vi "Post-Install Custom Action - Platform Specific PPLs.vi"(10 "Variant":variant) -> (0 "error out":errorcluster)   [LabVIEW 2020]
uses:
  <vilib>/Utility/lvfile.llb/FT_FileTypes.ctl
  <vilib>/Utility/lvfile.llb/NI_FileType.lvlib
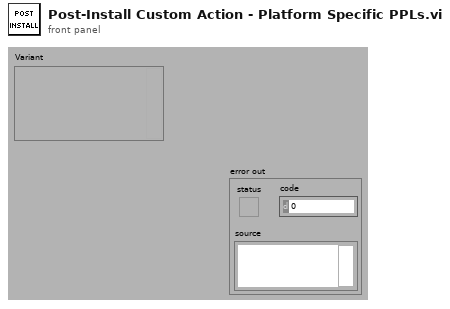
[diagram p1: front panel]
types:
  T1 = typedef "NI_FileType.lvlib/FT_FileTypes.ctl" = enum32{"Invalid file/path", "Unknown type", "Instrument", "Control", "Polymorphic VI", "Project", "Library", "LVClass", "XControl", "XNode", "CIN", "Run-time menu", "Palette menu", "LLB", "Shortcut", "Directory", "Class Private Data Control", "Statechart", "MathScript .m file", "Ladder Diagram", "LVLibp"}
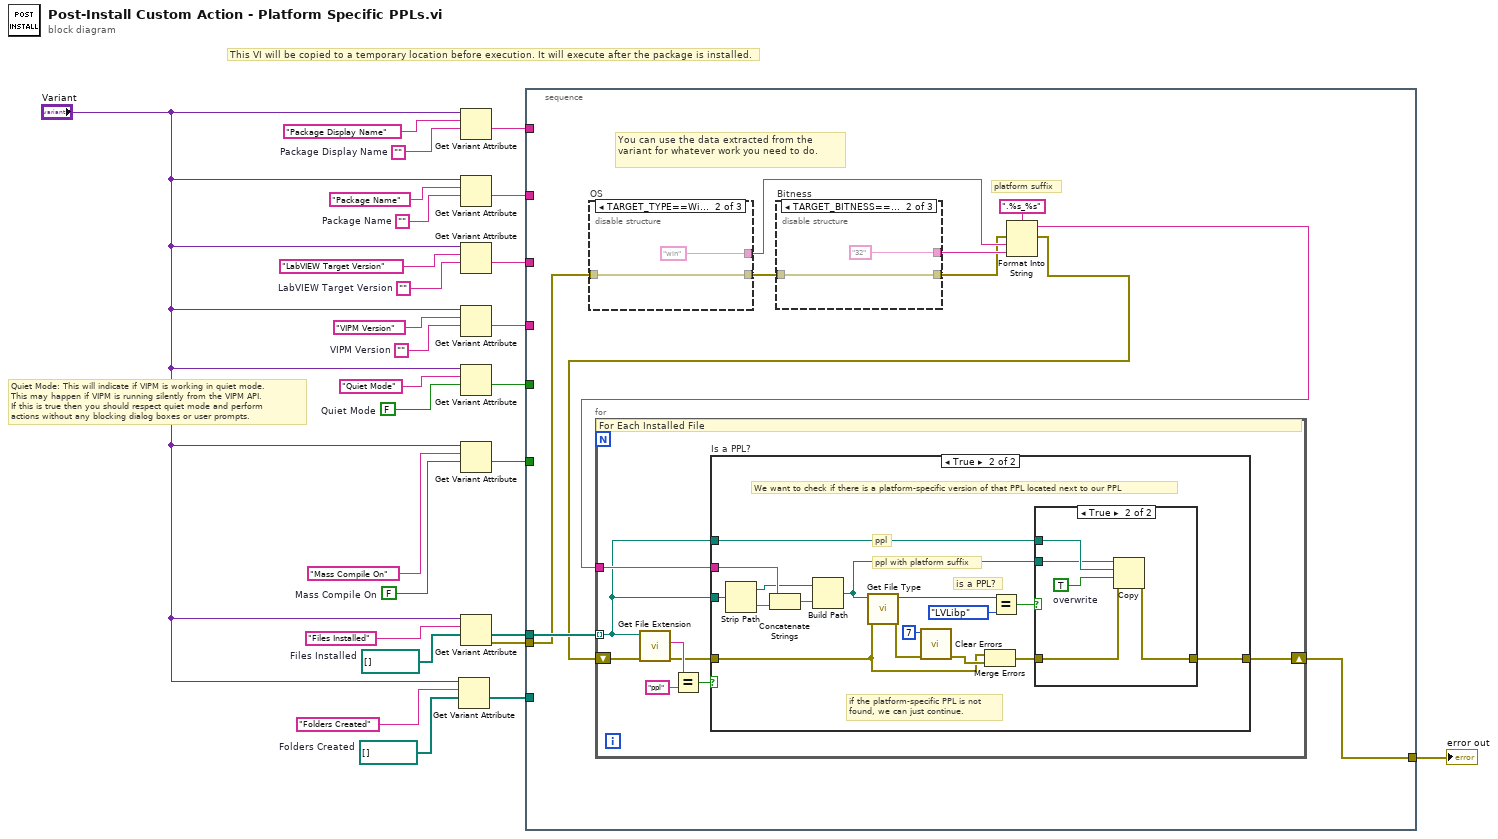
[diagram p0: block diagram]
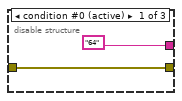
[diagram p2: hidden frame]
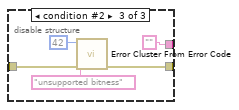
[diagram p3: hidden frame]
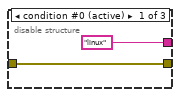
[diagram p4: hidden frame]
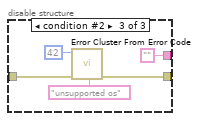
[diagram p5: hidden frame]
diagram:
  w3 = path[] []  # Folders Created
  w4 = path[] []  # Files Installed
  w10 = FALSE  # Mass Compile On
  w11 = ""  # Package Display Name
  w18 = FALSE  # Quiet Mode
  w21 = ""  # VIPM Version
  w23 = ""  # LabVIEW Target Version
  w25 = ""  # Package Name
  # "Quiet Mode: This will indicate if VIPM is working in quiet mode.\nThis may happen if VIPM is running silently from the VIPM API.\nIf this is true then you should respect quiet mode and perform\nactions without any blocking dialog boxes or user prompts."
  # "This VI will be copied to a temporary location before execution. It will execute after the package is installed."
  n1 = Get Variant Attribute(Variant="Variant", name="Folders Created", default value (empty Variant)=w3) -> (value=w8:path[])  [unwired: 1 in, 3 out]
  n2 = Get Variant Attribute(Variant="Variant", name="Package Display Name", default value (empty Variant)=w11) -> (value=w17:string)  [unwired: 1 in, 3 out]
  n3 = Get Variant Attribute(Variant="Variant", name="Package Name", default value (empty Variant)=w25) -> (value=w16:string)  [unwired: 1 in, 3 out]
  n4 = Get Variant Attribute(Variant="Variant", name="LabVIEW Target Version", default value (empty Variant)=w23) -> (value=w15:string)  [unwired: 1 in, 3 out]
  n5 = Get Variant Attribute(Variant="Variant", name="VIPM Version", default value (empty Variant)=w21) -> (value=w14:string)  [unwired: 1 in, 3 out]
  n6 = Get Variant Attribute(Variant="Variant", name="Quiet Mode", default value (empty Variant)=w18) -> (value=w13:bool)  [unwired: 1 in, 3 out]
  n7 = Get Variant Attribute(Variant="Variant", name="Mass Compile On", default value (empty Variant)=w10) -> (value=w12:bool)  [unwired: 1 in, 3 out]
  n8 = Get Variant Attribute(Variant="Variant", name="Files Installed", default value (empty Variant)=w4) -> (value=w7:path[], error out=w2:errorcluster)  [unwired: 1 in, 2 out]
  n9 = stacked-sequence {
    tunnel: w17 -> [_]
    tunnel: w16 -> [_]
    tunnel: w15 -> [_]
    tunnel: w14 -> [_]
    tunnel: w13 -> [_]
    tunnel: w12 -> [_]
    tunnel: w7 -> [w37]
    tunnel: w8 -> [_]
    tunnel: w2 -> [w35]
    tunnel: [w30] -> w1
    frame #0 {
      # "platform suffix"
      # "You can use the data extracted from the variant for whatever work you need to do."
      n10 = disable-structure "OS" shown="TARGET_TYPE==Windows" {
        disable-tunnel: ["linux" "win" ""] -> w34
        disable-tunnel: [w47 w49 w52] -> w36
        disable-tunnel: w35 -> [w47 w49 w51]
        frame condition #0 (active) {
        }
        frame condition #1 {
        }
        frame condition #2 {
          n11 = call <vilib>:"Error Cluster From Error Code.vi"("error in (no error)"=w51, "error message (\"\")"="unsupported os" ("error message (\"\")"), "error code (0)"=42) -> ("error out"=w52:errorcluster)  [unwired: 6 in]
        }
      }
      n12 = disable-structure "Bitness" shown="TARGET_BITNESS==32" {
        disable-tunnel: ["64" "32" ""] -> w33
        disable-tunnel: w36 -> [w38 w40 w43]
        disable-tunnel: [w38 w40 w42] -> w29
        frame condition #0 (active) {
        }
        frame condition #1 {
        }
        frame condition #2 {
          n13 = call <vilib>:"Error Cluster From Error Code.vi"("error in (no error)"=w43, "error message (\"\")"="unsupported bitness" ("error message (\"\")"), "error code (0)"=42) -> ("error out"=w42:errorcluster)  [unwired: 6 in]
        }
      }
      n14 = Format Into String(format string=".%s_%s", error in=w29, w34, w33) -> (resulting string=w31:string, error out=w28:errorcluster)  [unwired: 1 in]
      n15 = for {
        tunnel: w37 -> [w56] mode=indexing
        tunnel: w31 -> [w61]
        shift-right: [w57] -> w30
        shift-left: w28 -> [w58]
        # "For Each Installed File"
        n16 = call <vilib>:"Get File Extension.vi"("error in (no error)"=w58, "file"=w56) -> ("error out"=w59:errorcluster, "lowercase file extension"=w63:string)  [unwired: 5 in, 3 out]
        n17 = Equal?(x=w63, y="ppl" ("lowercase file extension")) -> (x = y?=w60:bool)
        n18 = case "Is a PPL?" shown="True" w60 {
          tunnel: w56 -> [_ w80]
          tunnel: w61 -> [_ w78]
          tunnel: w59 -> [w64 w69]
          tunnel: [w64 w68] -> w57
          tunnel: w56 -> [_ w66]
          frame False {
          }
          frame True {
            # "We want to check if there is a platform-specific version of that PPL located next to our PPL"
            # "is a PPL?"
            # "ppl"
            # "ppl with platform suffix"
            # "if the platform-specific PPL is not found, we can just continue."
            n19 = Strip Path(path=w80) -> (stripped path=w77:path, name=w79:string)
            n20 = Concatenate Strings(w78, w79) -> (w76:string)
            n21 = Build Path(base path=w77, name or relative path=w76) -> (appended path=w65:path)
            n22 = call <vilib>:"Get File Type.vi"("error in (no error)"=w69, "path"=w65) -> ("error out"=w72:errorcluster, "file type"=w74:T1)  [unwired: 7 in, 1 out]
            n23 = call <vilib>:"Clear Errors.vi"("error in (no error)"=w72, "specific error code to clear (0: all)"=7) -> ("error out"=w70:errorcluster)  [unwired: 4 in, 1 out]
            n24 = Merge Errors(w69, w70) -> (w67:errorcluster)
            n25 = Equal?(x=w74, y=FT_FileTypes."LVLibp" ("file type")) -> (x = y?=w73:bool)
            n26 = case shown="True" w73 {
              tunnel: [w81 w84] -> w68
              tunnel: w67 -> [w81 w83]
              tunnel: w66 -> [_ w86]
              tunnel: w65 -> [_ w85]
              frame False {
              }
              frame True {
                w82 = TRUE  # overwrite
                n27 = Copy(8:w83, 9:w82, 10:w86, 11:w85) -> (0:w84:errorcluster)  [unwired: 1 in, 2 out]
              }
            }
          }
        }
      }
    }
  }
  "error out" <- w1
